vi "oa_Compute RMS Overall Level.vi"(7 "reset":bool, 8 "integration revolution":dbl=1.0, 10 "even angle position info in":T1, 11 "even angle signals":cluster{"r0":dbl, "dr":dbl, "Y":dbl[]}[](array[cluster])) -> (0 "output length":i32, 1 "decimation factor":i32, 2 "even angle position info out":T1, 3 "output RMS level":dbl[][](array[numeric]))   [LabVIEW 2017, in "SoundVib_Resampling.lvlib"]
uses:
  <vilib>/addons/Sound and Vibration/Order Analysis/Resample Order Tracking/SoundVib_Resampling.lvlib
  <vilib>/addons/Sound and Vibration/Order Analysis/Misc/OAT Position Info.ctl
  <vilib>/Analysis/5stat.llb/RMS (DBL).vi
  <vilib>/Analysis/NI_AALPro.lvlib
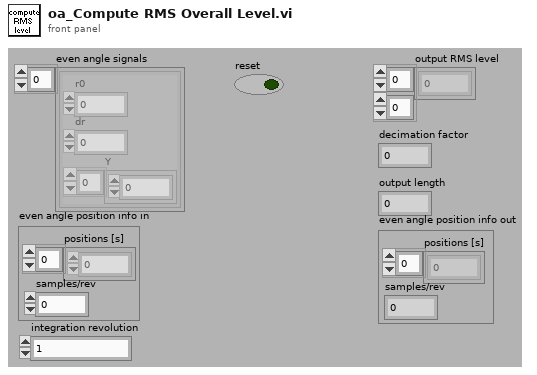
[diagram p1: front panel]
types:
  T1 = typedef "OAT Position Info.ctl" = cluster{"positions [s]":dbl[], "samples/rev":dbl}
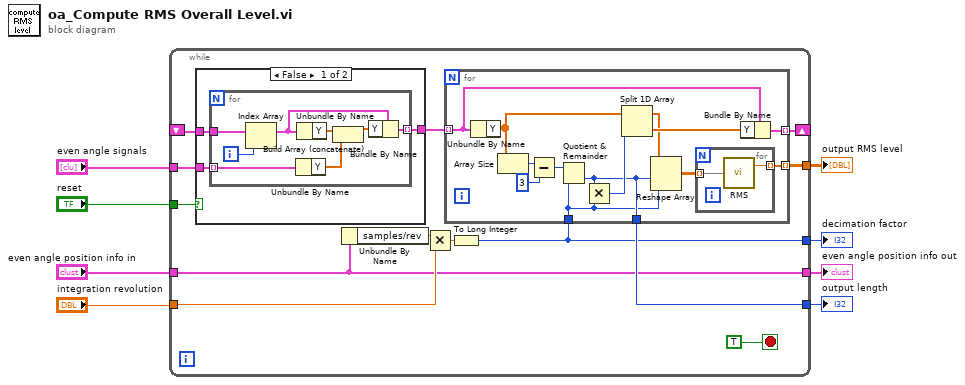
[diagram p0: block diagram]
diagram:
  n1 = while {
    tunnel: "integration revolution" -> [w10]
    tunnel: "even angle signals" -> [w19]
    tunnel: "reset" -> [w18]
    shift-right: [w15] -> _
    shift-left: _ -> [w20]
    tunnel: "even angle position info in" -> [w9]
    tunnel: [w14] -> w7
    tunnel: [w11] -> w8
    tunnel: [w12] -> w6
    tunnel: [w9] -> w1
    stop <- TRUE stop-if-true
    n2 = case shown="False" w18 {
      tunnel: w20 -> [w39 _]
      tunnel: w19 -> [w38 w48]
      tunnel: [w37 w48] -> w17
      frame False {
        n3 = for {
          tunnel: w39 -> [w46]
          tunnel: w38 -> [w47] mode=indexing
          tunnel: [w43] -> w37 mode=indexing
          i -> [w40]
          n4 = Index Array(array=w46, index=w40) -> (element=w41:cluster{"r0":dbl, "dr":dbl, "Y":dbl[]})
          n5 = Unbundle By Name(w47) -> ("Y"=w44:dbl[])
          n6 = Unbundle By Name(w41) -> ("Y"=w45:dbl[])
          n7 = Build Array (concatenate)(w45, w44) -> (w42:dbl[])
          n8 = Bundle By Name(cluster=w41, "Y"=w42) -> (w43:cluster{"r0":dbl, "dr":dbl, "Y":dbl[]})
        }
      }
      frame True {
      }
    }
    n9 = Unbundle By Name(w9) -> ("samples/rev"=w16:dbl)
    n10 = Multiply(x=w16, y=w10) -> (x*y=w13:dbl)
    n11 = To Long Integer(number=w13) -> (32bit integer=w11:i32)
    n12 = for {
      tunnel: w17 -> [w34] mode=indexing
      tunnel: w11 -> [w25]
      tunnel: [w33] -> w15 mode=indexing
      tunnel: [w29] -> w14 mode=indexing
      tunnel: [w26] -> w12
      n13 = Unbundle By Name(w34) -> ("Y"=w31:dbl[])
      n14 = Array Size(array=w31) -> (size(s)=w32:i32)
      n15 = Subtract(x=w32, y=3) -> (x-y=w23:i32)
      n16 = Quotient & Remainder(x=w23, y=w25) -> (floor(x/y)=w26:i32)  [unwired: 1 out]
      n17 = Multiply(x=w26, y=w25) -> (x*y=w30:i32)
      n18 = Split 1D Array(array=w31, index=w30) -> (first subarray=w27:dbl[], second subarray=w28:dbl[])
      n19 = Reshape Array(w27, w26, w25) -> (w24:dbl[][])
      n20 = for {
        tunnel: [w36] -> w29 mode=indexing
        tunnel: w24 -> [w35] mode=indexing
        n21 = call-poly <vilib>:"RMS.vi"("X"=w35) -> ("rms value"=w36:dbl)  [unwired: 1 out]
      }
      n22 = Bundle By Name(cluster=w34, "Y"=w28) -> (w33:cluster{"r0":dbl, "dr":dbl, "Y":dbl[]})
    }
  }
  "decimation factor" <- w8
  "output RMS level" <- w7
  "output length" <- w6
  "even angle position info out" <- w1
